vi "Reset Encoder.vi"() -> ()   [LabVIEW 2016]
panel:
  out "Auto Encoder reset":bool
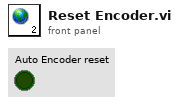
[diagram p1: front panel]
diagram:
